vi "BRig_dataExp_T_Cue2_LED_max.vi"() -> (2 "output_T_Cue2_LED_max":i32)   [LabVIEW 2014]
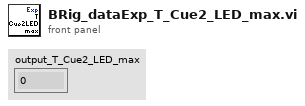
[diagram p1: front panel]
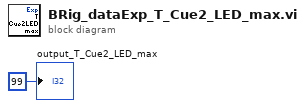
[diagram p0: block diagram]
diagram:
  "output_T_Cue2_LED_max" <- 99 ("output_iBlock")
